vi "SplitGCode.vi"(2 "error in":errorcluster, 3 "string":string) -> (0 "error out":errorcluster, 1 "Cluster":T1)   [LabVIEW 2016]
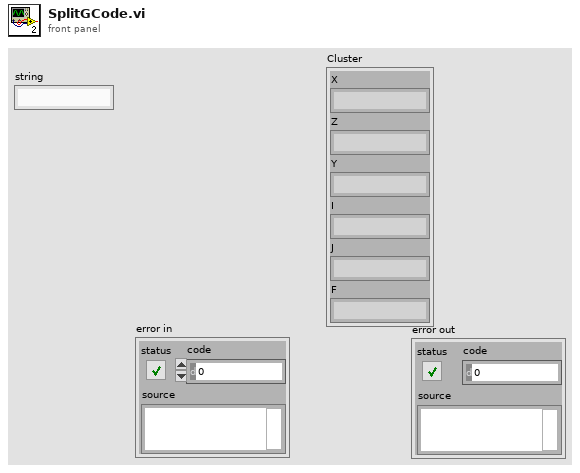
[diagram p1: front panel]
types:
  T1 = cluster{"X":string, "Z":string, "Y":string, "I":string, "J":string, "F":string}
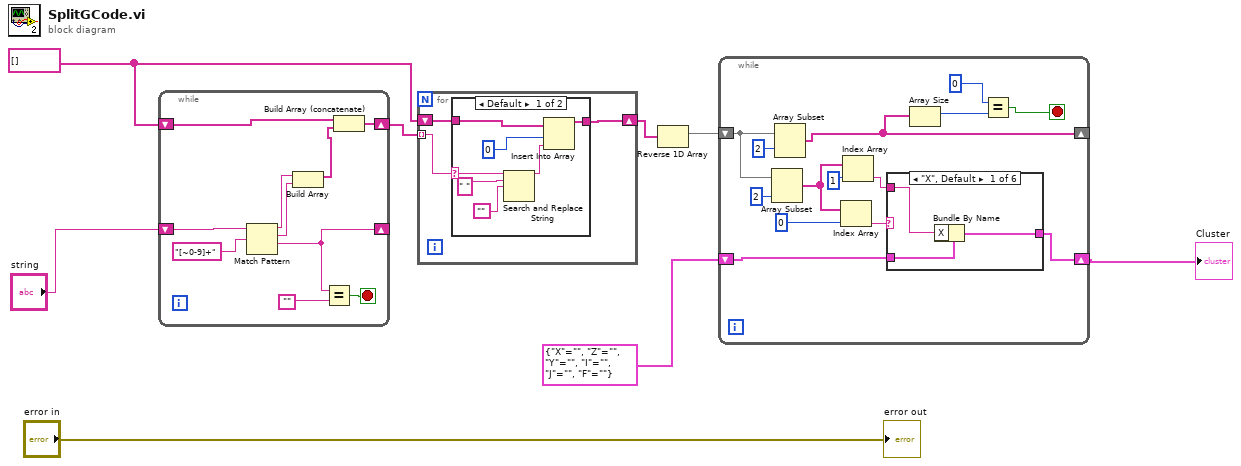
[diagram p0: block diagram]
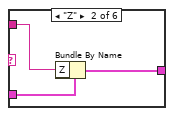
[diagram p2: hidden frame]
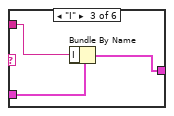
[diagram p3: hidden frame]
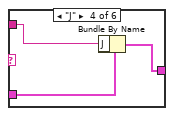
[diagram p4: hidden frame]
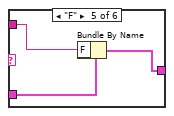
[diagram p5: hidden frame]
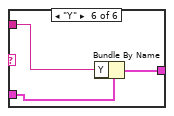
[diagram p6: hidden frame]
diagram:
  w6 = string[] []
  n1 = while {
    shift-right: [w14] -> _
    shift-left: "string" -> [w17]
    shift-right: [w11] -> w7
    shift-left: w6 -> [w10]
    stop <- w15 stop-if-true
    n2 = Match Pattern(string=w17, regular expression="[~0-9]+") -> (before substring=w13:string, match substring=w12:string, after substring=w14:string)  [unwired: 1 in, 1 out]
    n3 = Build Array(w13, w12) -> (w9:string[])
    n4 = Equal?(x=w14, y="") -> (x = y?=w15:bool)
    n5 = Build Array (concatenate)(w10, w9) -> (w11:string[])
  }
  n6 = for {
    tunnel: w7 -> [w21] mode=indexing
    shift-right: [w19] -> w5
    shift-left: w6 -> [w20]
    n7 = case shown="Default" w21 {
      selector: w21 -> [w25 _]
      tunnel: w20 -> [w28 w29]
      tunnel: [w27 w29] -> w19
      frame Default {
        n8 = Search and Replace String(input string=w25, search string=" ", replace string="") -> (result string=w22:string)  [unwired: 5 in, 3 out]
        n9 = Insert Into Array(array=w28, index=0, new element=w22) -> (w27:string[])
      }
      frame "" {
      }
    }
  }
  n10 = Reverse 1D Array(array=w5) -> (reversed array=w4:string[])
  n11 = while {
    shift-right: [w37] -> _
    shift-left: w4 -> [w31]
    shift-right: [w39] -> w1
    shift-left: T1 {"X"="", "Z"="", "Y"="", "I"="", "J"="", "F"=""} -> [w38]
    stop <- w36 stop-if-true
    n12 = Array Subset(array=w31, length=2) -> (w30:string[])  [unwired: 1 in]
    n13 = Array Subset(array=w31, index=2) -> (w37:string[])  [unwired: 1 in]
    n14 = Index Array(array=w30, index=0) -> (element=w41:string)
    n15 = Index Array(array=w30, index=1) -> (element=w43:string)
    n16 = case shown="\"X\", Default" w41 {
      tunnel: w43 -> [w44 w47 w52 w55 w58 w61]
      tunnel: w38 -> [w46 w48 w51 w54 w57 w60]
      tunnel: [w45 w49 w50 w53 w56 w59] -> w39
      frame "X", Default {
        n17 = Bundle By Name(cluster=w46, "X"=w44) -> (w45:T1)
      }
      frame "Z" {
        n18 = Bundle By Name(cluster=w48, "Z"=w47) -> (w49:T1)
      }
      frame "I" {
        n19 = Bundle By Name(cluster=w51, "I"=w52) -> (w50:T1)
      }
      frame "J" {
        n20 = Bundle By Name(cluster=w54, "J"=w55) -> (w53:T1)
      }
      frame "F" {
        n21 = Bundle By Name(cluster=w57, "F"=w58) -> (w56:T1)
      }
      frame "Y" {
        n22 = Bundle By Name(cluster=w60, "Y"=w61) -> (w59:T1)
      }
    }
    n23 = Array Size(array=w37) -> (size(s)=w35:i32)
    n24 = Equal?(x=0, y=w35) -> (x = y?=w36:bool)
  }
  "Cluster" <- w1
  "error out" <- "error in"
